vi "Fetch Interface Documentation.vi"(8 "error in (no error)":errorcluster {"code" format="Error %.0f"}, 10 "Parser Settings":T1, 11 "Interface in":refnum<vi>) -> (0 "error out":errorcluster {"code" format="Error %.0f"}, 3 "Interface Documenation Out":refnum<class "Interface Documenation.lvclass">)   [LabVIEW 2023, in "VIDoc Parsing.lvlib" / "Interface Documenation.lvclass"]
doc: "Takes an Interface Reference in and parses out all Interface Documentation information needed for document generation."
uses:
  Interface Documenation.lvclass
  Settings/Parser Settings/Parser Settings Cluster.ctl
  Settings/Parser Settings/Draw Controls Cluster.ctl
  Settings/Parser Settings/Draw Option Enum.ctl
  Interface Documenation.lvclass/Interface Documenation.ctl
  VIDoc Parsing.lvlib
  Settings/Parser Settings/Parser Settings.lvclass
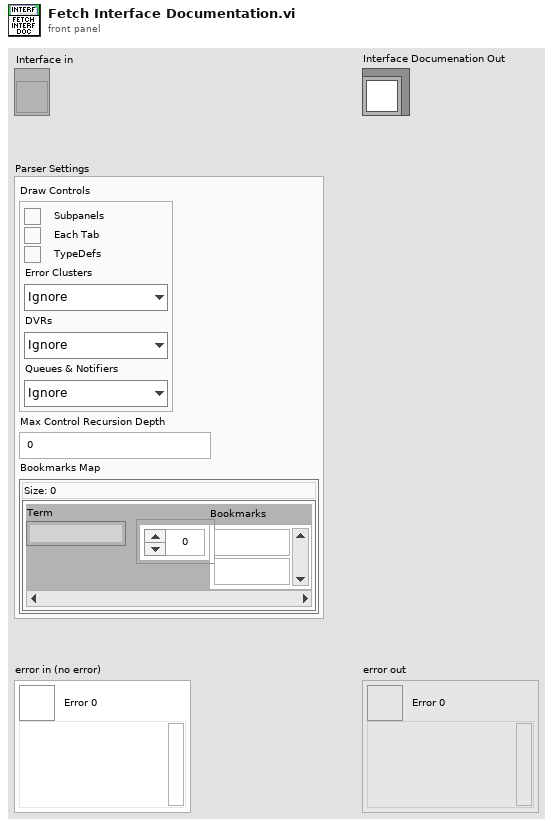
[diagram p1: front panel]
types:
  T1 = typedef "VIDoc Parsing.lvlib/Parser Settings.lvclass/Parser Settings Cluster.ctl" = cluster{"Draw Controls":T2, "Max Control Recursion Depth":i32, "Bookmarks Map":map{string, string[]}}
  T2 = typedef "VIDoc Parsing.lvlib/Parser Settings.lvclass/Draw Controls Cluster.ctl" = cluster{"Subpanels":bool, "Tabs":bool, "TypeDefs":bool, "Error Clusters":T3, "DVRs":T3, "Queues & Notifiers":T3}
  T3 = typedef "VIDoc Parsing.lvlib/Parser Settings.lvclass/Draw Option Enum.ctl" = enum16{"Ignore", "Draw", "Draw + Contents"}
  T4 = typedef "VIDoc Parsing.lvlib/Base Class Info Cluster.ctl" = cluster{"Name":string, "Icon":T5, "Version":cluster{"Major":u16, "Minor":u16, "Fix":u16, "Build":u16}, "Description":string, "Friends":string[], "ChildRefsRestricted":bool, "TransferMustOverrides":bool, "Path":path, "Qualified Name":string, "Class Scope":enum32{"invalid scope", "public", "private", "protected", "community"}}
  T5 = typedef "imagedata.ctl" = cluster{"image type":i32, "image depth":i32, "image":u8[], "mask":u8[], "colors":u32[], "Rectangle":cluster{"left":i16, "top":i16, "right":i16, "bottom":i16}}
  T6 = typedef "VIDoc Parsing.lvlib/Method Spec Cluster.ctl" = cluster{"VI Type Ext":T7, "Name":string, "Path":path, "Get Conpane Image":T5, "Description":string, "Get Library Access Scope":enum32{"invalid scope", "public", "private", "protected", "community"}, "Dispatch":T8, "ContainsCompiledCode":bool, "Exec.IsReentrant":bool, "Exec.ReentrancyType":enum16{"Share clones between instances", "Preallocate clone for each instance"}, "ExecInlining":bool, "ExecInlineIfPossible":bool, "Auto Err Handling":bool, "CodeComplexity":sgl, "Bookmark Tags":string[], "Control VI Type":enum32{"not a control VI", "control", "typedef", "strict typedef"}, "Controls":T9[], "VI Type":enum32{"invalid VI type", "Standard VI", "Control VI", "Global VI", "Polymorphic VI", "Configuration VI", "SubSystem", "Facade VI", "Method VI", "Statechart Diagram VI"}, "Minimum Size":T11, "Front Panel Window:Title":string, "Front Panel Window:Behavior":enum32{"Invalid", "Default", "Floating", "Floating/Auto-Hide", "Modal"}, "Front Panel Window:Closeable":bool, "Must Override":bool, "Must Use Parent Implementation":bool, "VI Icon":T5, "Front Panel":T5, "History:Revision Number":u32, "Metrics:Total Data Size":u32, "Execution:Allow Debugging":bool, "Execution:Preferred Exec System":enum32{"invalid execution system", "user interface", "standard", "instrument i/o", "data acquisition", "other 1", "other 2", "same as caller"}, "Execution:Priority":enum32{"invalid priority", "background priority", "normal priority", "above normal priority", "high priority", "time critical priority", "subroutine"}, "BM Tag Text":string[], "Block Diagram":T5, "Structure Tree":T12[]}
  T7 = typedef "VIDoc Parsing.lvlib/VI Type Extended Enum.ctl" = enum16{"Unknown", "Class Method", "Class Accessor Get", "Class Accessor Set", "Class Control", "Library Method", "Library Control", "VI", "Control"}
  T8 = typedef "VIDoc Parsing.lvlib/Class Dispatch Type Enum.ctl" = enum16{"None", "Static", "Dynamic"}
  T9 = typedef "VIDoc Parsing.lvlib/Controls Info Cluster.ctl" = cluster{"Name":string, "Description":string, "Data Type":string, "Tip Strip":string, "UID":i32, "Image Data":T5, "ToggleKeyBind":T10, "Raw Label":string, "Raw Caption":string}
  T10 = typedef "LVKeyTypeDef.ctl" = cluster{"Focus":bool, "Control":bool, "Shift":bool, "Key":string}
  T11 = typedef "LVPointTypeDef.ctl" = cluster{"Horizontal":i16, "Vertical":i16}
  T12 = typedef "VIDoc Parsing.lvlib/Structure Reporter.lvlib/Tree Cluster.ctl" = cluster{"Object Class Name":string, "Labels":string[], "Child Tag":string, "Item Indent":i32, "Child Only?":bool, "Glyph Index":i32}
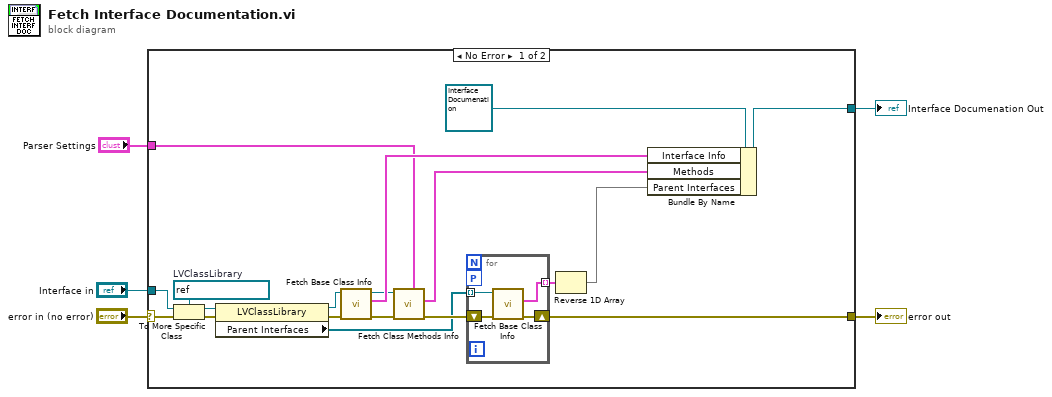
[diagram p0: block diagram]
diagram:
  n1 = case shown="No Error" "error in (no error)" {
    selector: "error in (no error)" -> [w23 w29]
    tunnel: [w9 w29] -> w4
    tunnel: "Interface in" -> [w22 _]
    tunnel: [w20 _] -> w2
    tunnel: "Parser Settings" -> [w15 _]
    frame No Error {
      w24 = refnum<vi> refnum  # LVClassLibrary
      n2 = To More Specific Class(target class=w24, reference=w22, error in=w23) -> (specific class reference=w12:refnum<vi>, error out=w14:errorcluster)
      n3 = property class="LVClassLibrary"(reference=w12, error in=w14) -> (reference out=w11:refnum<vi>, error out=w13:errorcluster, "Parent Interfaces"=w8:refnum<vi>[])
      n4 = call "Fetch Base Class Info.vi"("error in (no error)"=w13, "LVClassLibrary in"=w11) -> ("error out"=w17:errorcluster, "Base Class Info"=w19:T4, "LVClassLibrary out"=w18:refnum<vi>)  [unwired: 7 in]
      n5 = call "Fetch Class Methods Info.vi"("Parser Settings"=w15, "Error in"=w17, "LVClassLibrary"=w18) -> ("Error out"=w10:errorcluster, "Methods"=w16:T6[])  [unwired: 7 in]
      n6 = for {
        tunnel: [w26] -> w7 mode=indexing
        tunnel: w8 -> [w27] mode=indexing
        shift-right: [w25] -> w9
        shift-left: w10 -> [w28]
        workers-P: _ -> [_]
        n7 = call "Fetch Base Class Info.vi"("error in (no error)"=w28, "LVClassLibrary in"=w27) -> ("error out"=w25:errorcluster, "Base Class Info"=w26:T4)  [unwired: 7 in, 1 out]
      }
      n8 = Reverse 1D Array(array=w7) -> (reversed array=w6:T4[])
      n9 = Bundle By Name(cluster=refnum<class "Interface Documenation.lvclass"> refnum ("Interface Documenation out"), "Interface Info"=w19, "Methods"=w16, "Parent Interfaces"=w6) -> (w20:refnum<class "Interface Documenation.lvclass">)
    }
    frame Error {
    }
  }
  "error out" <- w4
  "Interface Documenation Out" <- w2
